vi "ROS_Service_Setup.vi"(3 "Specs":T3={"Server"="", "Node"="/labview", "Server Port"=5000, "URI (Subsc)"="", "connection"=refnum, "Direction"=enum."Node"}, 4 "Msg to Send":string, 5 "Requests In":T1(array[cluster])) -> (0 "error out":errorcluster, 1 "Reply":string, 2 "Requests Out":T1(array[cluster]))   [LabVIEW 2010]
doc: "Creates and sends the connection header and message to a service provider. Implemented in the background server."
uses:
  <userlib>/ROSforLV_0.1/ROS/Code/SubVIs/_ROSDirection.ctl
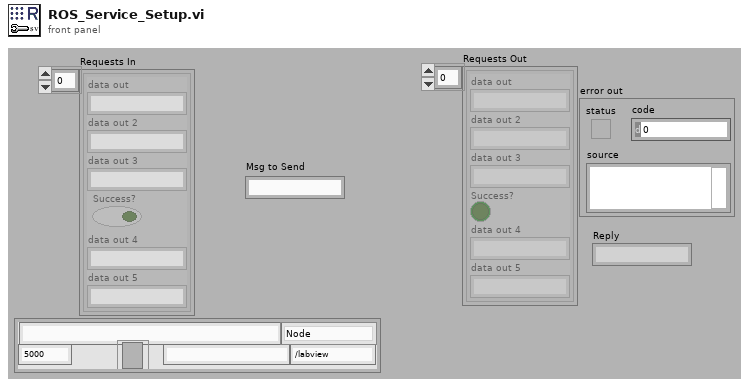
[diagram p1: front panel]
types:
  T1 = cluster{"data out":string, "data out 2":string, "data out 3":string, "Success?":bool, "data out 4":string, "data out 5":string}[]
  T2 = typedef "_ROSDirection.ctl" = enum16{"Node", "Publisher", "Subscriber", "Service Client"}
  T3 = cluster{"Server":string, "Node":string, "Server Port":u32, "URI (Subsc)":string, "connection":refnum<k5>, "Direction":T2}
  T4 = cluster{"data out":string, "data out 2":string, "data out 3":string, bool, "data out 4":string, "data out 5":string}
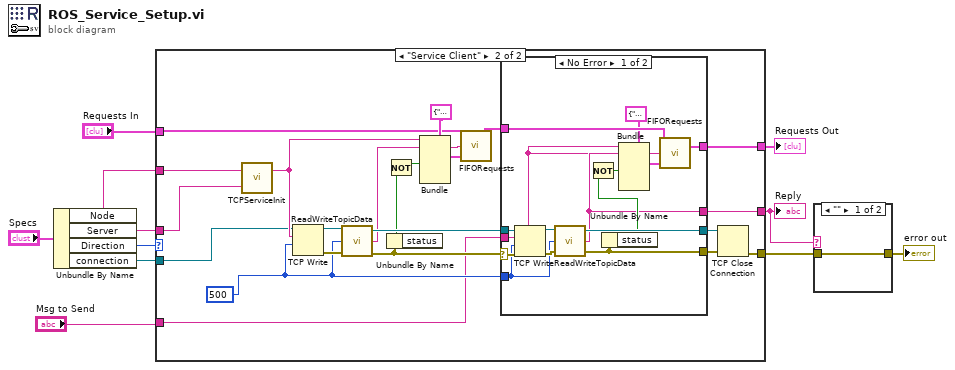
[diagram p0: block diagram]
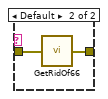
[diagram p2: hidden frame]
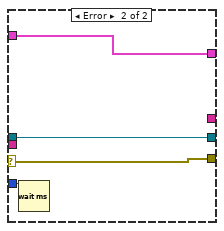
[diagram p4: hidden frame]
diagram:
  n1 = Unbundle By Name("Specs") -> ("Node"=w9:string, "Server"=w8:string, "Direction"=w10:T2, "connection"=w1:refnum<k5>)
  n2 = case shown="\"Service Client\"" w10 {
    tunnel: w9 -> [_ w26]
    tunnel: w8 -> [_ w25]
    tunnel: "Requests In" -> [w12 w24]
    tunnel: [w12 w16] -> w6
    tunnel: [_ w18] -> w3
    tunnel: "Msg to Send" -> [_ w15]
    tunnel: [_ w14] -> w4
    tunnel: w1 -> [_ w13]
    frame Default {
    }
    frame "Service Client" {
      w27 = 500 ("timeout ms (60000)")
      n3 = call <userlib>:"TCPServiceInit.vi"("topic"=w25, "callerID"=w26) -> ("TCP ROS Reply"=w31:string)  [unwired: 1 out]
      n4 = TCP Write(connection ID=w13, data in=w31, 9:w27) -> (connection ID out=w34:refnum<k5>, error out=w33:errorcluster)  [unwired: 1 in, 1 out]
      n5 = call <userlib>:"ReadWriteTopicData.vi"("error in (no error)"=w33, "timeout ms (1000)"=w27, "connection ID in"=w34) -> ("error out"=w22:errorcluster, "data out"=w29:string, "connection ID out"=w32:refnum<k5>)
      n6 = Unbundle By Name(w22) -> ("status"=w21:bool)
      n7 = Not(x=w21) -> (.not. x?=w20:bool)
      n8 = Bundle(cluster=T4 {"data out"="", "data out 2"="", "data out 3"="subscriber", FALSE, "data out 4"="To Baxter", "data out 5"="From Baxter"}, "data out"=w31, "data out 2"=w29, w20) -> (w30:T4)  [unwired: 3 in]
      n9 = call <userlib>:"FIFORequests.vi"("New One"=w30, "data out"=w29, "Requests In"=w24) -> ("Requests Out"=w17:T1)
      n10 = case shown="No Error" w22 {
        selector: w22 -> [w45 w51]
        tunnel: w32 -> [w47 w52]
        tunnel: w27 -> [w35 w53]
        tunnel: [w46 w52] -> w23
        tunnel: [w40 w51] -> w19
        tunnel: w17 -> [w43 w50]
        tunnel: [w42 w50] -> w16
        tunnel: w15 -> [w36 _]
        tunnel: [w37 _] -> w14
        frame No Error {
          n11 = TCP Write(connection ID=w47, data in=w36, error in (no error)=w45, 9:w35) -> (connection ID out=w49:refnum<k5>, error out=w48:errorcluster)  [unwired: 1 out]
          n12 = call <userlib>:"ReadWriteTopicData.vi"("error in (no error)"=w48, "timeout ms (1000)"=w35, "connection ID in"=w49) -> ("error out"=w40:errorcluster, "data out"=w37:string, "connection ID out"=w46:refnum<k5>)
          n13 = Unbundle By Name(w40) -> ("status"=w39:bool)
          n14 = Not(x=w39) -> (.not. x?=w38:bool)
          n15 = Bundle(cluster=T4 {"data out"="", "data out 2"="", "data out 3"="write", FALSE, "data out 4"="To Baxter", "data out 5"="From Baxter"}, "data out"=w36, "data out 2"=w37, w38) -> (w44:T4)  [unwired: 3 in]
          n16 = call <userlib>:"FIFORequests.vi"("New One"=w44, "data out"=w36, "Requests In"=w43) -> ("Requests Out"=w42:T1)
        }
        frame Error {
          n17 = Wait (ms)(milliseconds to wait=w53) -> ()  [unwired: 1 out]
        }
      }
      n18 = TCP Close Connection(connection ID=w23, error in (no error)=w19) -> (error out=w18:errorcluster)  [unwired: 1 in, 1 out]
    }
  }
  "Requests Out" <- w6
  "Reply" <- w4
  n19 = case shown="\"\"" w4 {
    tunnel: w3 -> [w54 w56]
    tunnel: [w54 w55] -> w2
    frame "" {
    }
    frame Default {
      n20 = call <userlib>:"GetRidOf66.vi"("error in (no error)"=w56) -> ("error out"=w55:errorcluster)
    }
  }
  "error out" <- w2
